vi "verificar_error_mbed.vi"(8 "error in (no error)":errorcluster, 10 "desde_mbed":string="AL") -> (0 "error out":errorcluster, 2 "error?":bool)   [LabVIEW 2011]
doc: "<b>MANEJO DE ERRORES:</b>\n\nSubVI dedicado al manejo de errores provenientes del microcontrolador ARM MBED. Esta función define errores y alarmas propios del deslizador:\n\n<b>AL:</b> Código 5001: Alarma desde el servodrive\n<b>A0:</b> Código 5002: Error, el deslizador se encuentra demasiado cerca al extremo del motor\n<b>A1:</b> Código 5003: Error, el deslizador se encuentra demasiado cerca al extremo del encoder\n<b>A2:</b> Código 5004: Alarma, el deslizador ha cruzado el limite en el extremo del motor\n<b>A3:</b> Código 5005: Alarma, el deslizador ha cruzado el limite en el extremo del encoder\n<b>A4:</b> Código 5006: Error, se ha enviado un comando no reconocido por el microcontrolador."
panel:
  # "Verifica e Imprime mensaje personalizado\nen caso de que el driver lo indique en la\nsalida ALM"
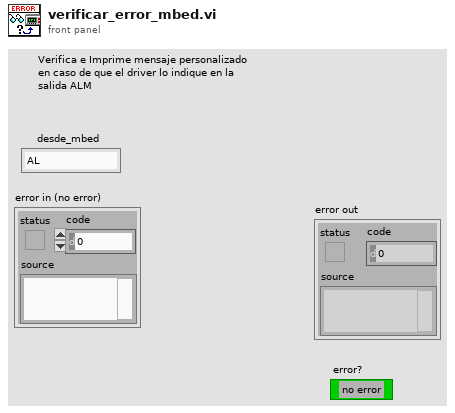
[diagram p1: front panel]
types:
  T1 = enum16{"ALM", "FIN CARRERA MOTOR", "ADVERT MOTOR", "ADVERT ENCODER", "FIN CARRERA ENC", "NUMERICO", "noError"}
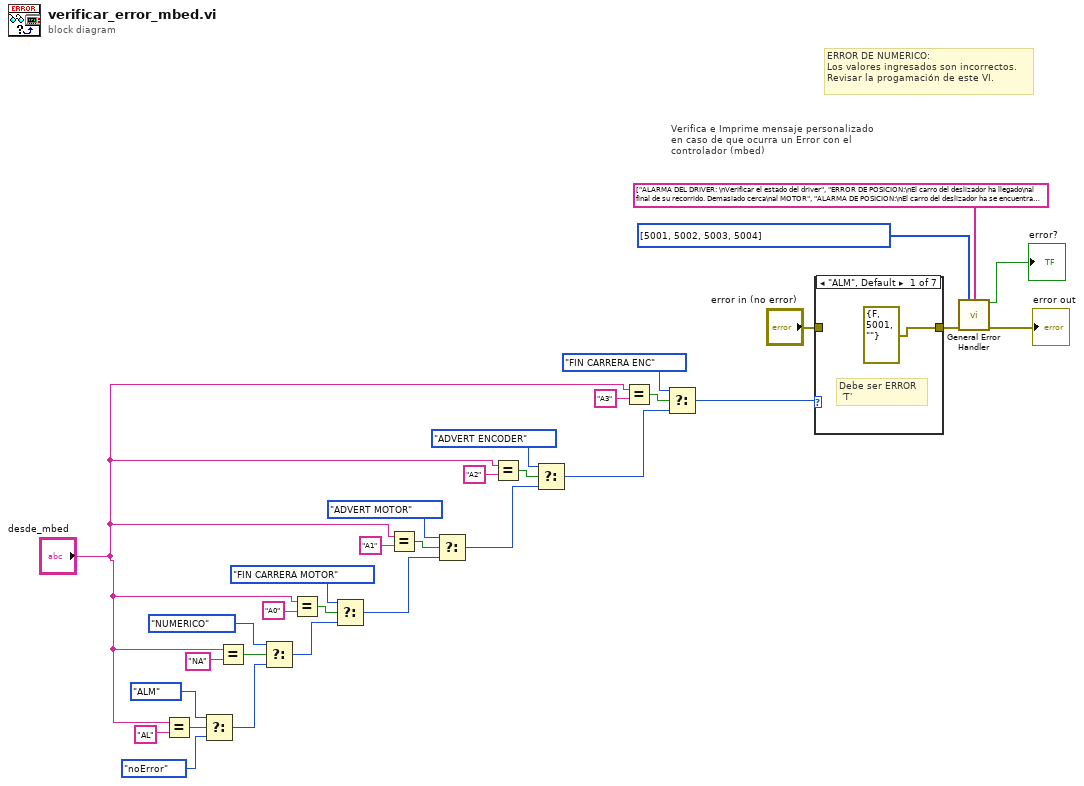
[diagram p0: block diagram]
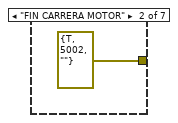
[diagram p2: hidden frame]
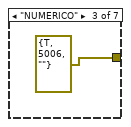
[diagram p3: hidden frame]
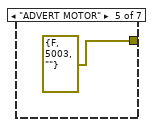
[diagram p5: hidden frame]
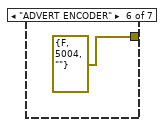
[diagram p6: hidden frame]
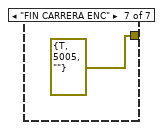
[diagram p7: hidden frame]
diagram:
  # "ERROR DE NUMERICO:\nLos valores ingresados son incorrectos.\nRevisar la progamación de este VI."
  # "Verifica e Imprime mensaje personalizado\nen caso de que ocurra un Error con el \ncontrolador (mbed)"
  n1 = Equal?(x="desde_mbed", y="AL") -> (x = y?=w25:bool)
  n2 = Select(t=T1."ALM", s=w25, f=T1."noError") -> (s? t:f=w22:T1)
  n3 = Equal?(x="desde_mbed", y="NA") -> (x = y?=w23:bool)
  n4 = Select(t=T1."NUMERICO", s=w23, f=w22) -> (s? t:f=w18:T1)
  n5 = Equal?(x="desde_mbed", y="A0") -> (x = y?=w20:bool)
  n6 = Select(t=T1."FIN CARRERA MOTOR", s=w20, f=w18) -> (s? t:f=w12:T1)
  n7 = Equal?(x="desde_mbed", y="A1") -> (x = y?=w14:bool)
  n8 = Select(t=T1."ADVERT MOTOR", s=w14, f=w12) -> (s? t:f=w9:T1)
  n9 = Equal?(x="desde_mbed", y="A2") -> (x = y?=w11:bool)
  n10 = Select(t=T1."ADVERT ENCODER", s=w11, f=w9) -> (s? t:f=w6:T1)
  n11 = Equal?(x="desde_mbed", y="A3") -> (x = y?=w8:bool)
  n12 = Select(t=T1."FIN CARRERA ENC", s=w8, f=w6) -> (s? t:f=w2:T1)
  n13 = case shown="\"ALM\", Default" w2 {
    tunnel: "error in (no error)" -> [_ _ _ w36 _ _ _]
    tunnel: [errorcluster {"status"=FALSE, "code"=5001, "source"=""} ("error out 2") errorcluster {"status"=TRUE, "code"=5002, "source"=""} ("error out 2") errorcluster {"status"=TRUE, "code"=5006, "source"=""} ("error out 2") w36 errorcluster {"status"=FALSE, "code"=5003, "source"=""} ("error out 2") errorcluster {"status"=FALSE, "code"=5004, "source"=""} ("error out 2") errorcluster {"status"=TRUE, "code"=5005, "source"=""} ("error out 2")] -> w28
    frame "ALM", Default {
      # "Debe ser ERROR \n 'T'"
    }
    frame "FIN CARRERA MOTOR" {
    }
    frame "NUMERICO" {
    }
    frame "noError" {
    }
    frame "ADVERT MOTOR" {
    }
    frame "ADVERT ENCODER" {
    }
    frame "FIN CARRERA ENC" {
    }
  }
  n14 = call <vilib>:"General Error Handler.vi"("[user-defined codes]"=i32[] [5001, 5002, 5003, 5004], "[user-defined descriptions]"=string[] ["ALARMA DEL DRIVER: \nVerificar el estado del driver", "ERROR DE POSICION:\nEl carro del deslizador ha llegado\nal final de su recorrido. Demasiado cerca\nal MOTOR", "ALARMA DE POSICION:\nEl carro del deslizador ha se encuentra demasiado cerca\nal final de su recorrido. MOTOR", "ALARMA DE POSICION:\nEl carro del deslizador ha se encuentra demasiado cerca\nal final de su recorrido. ENCODER", "ERROR DE POSICION:\nEl carro del deslizador ha llegado\nal final de su recorrido. Demasiado cerca\nal ENCODER", "ERROR DE POSICION: El comando enviado no ha sido reconocido.Por favor revise su programación."], "error in (no error)"=w28) -> ("error?"=→"error?":bool, "error out"=→"error out":errorcluster)  [unwired: 8 in, 3 out]
